vi "Application name.vi"() -> (0 "Ini file path":path, 1 "download site":string, 2 "help site":string, 3 "application name":string)   [LabVIEW 2010]
panel:
  out "Callers' Names":string[](array[string])
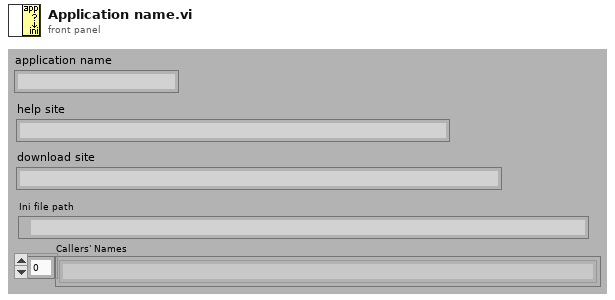
[diagram p1: front panel]
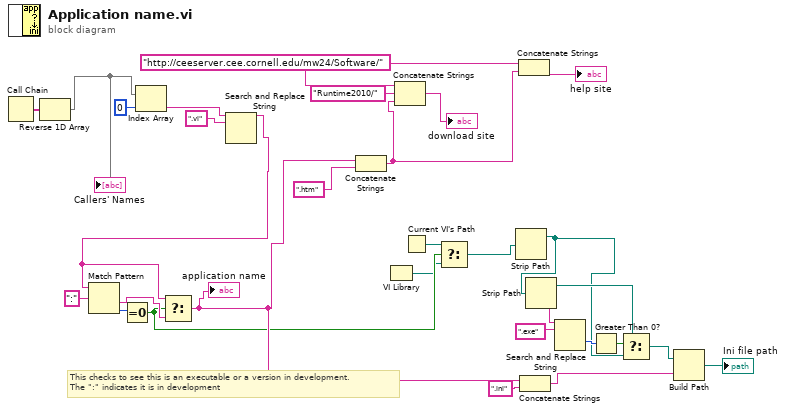
[diagram p0: block diagram]
diagram:
  w24 = "http://ceeserver.cee.cornell.edu/mw24/Software/"
  # "This checks to see this is an executable or a version in development.\nThe \":\" indicates it is in development"
  n1 = Call Chain() -> (call chain=w11:string[])
  n2 = Reverse 1D Array(array=w11) -> (reversed array=w10:string[])
  "Callers' Names" <- w10
  n3 = Index Array(array=w10, index=0) -> (element=w28:string)
  n4 = Search and Replace String(input string=w28, search string=".vi" ("replace string (\"\")")) -> (result string=w6:string)  [unwired: 6 in, 3 out]
  n5 = Match Pattern(string=w6, regular expression=":") -> (after substring=w7:string, offset past match=w8:i32)  [unwired: 1 in, 2 out]
  n6 = Equal To 0?(x=w8) -> (x = 0?=w4:bool)
  n7 = Select(t=w6, s=w4, f=w7) -> (s? t:f=w5:string)
  "application name" <- w5
  n8 = Concatenate Strings(w5, ".htm" ("replace string (\"\")")) -> (w22:string)
  n9 = VI Library() -> (path=w1:path)
  n10 = Concatenate Strings(w24, "Runtime2010/" ("string"), w22) -> (→"download site":string)
  n11 = Current VI's Path() -> (path=w3:path)
  n12 = Select(t=w3, s=w4, f=w1) -> (s? t:f=w2:path)
  n13 = Strip Path(path=w2) -> (stripped path=w16:path)  [unwired: 1 out]
  n14 = Concatenate Strings(w24, w22) -> (→"help site":string)
  n15 = Concatenate Strings(w5, ".ini") -> (w13:string)
  n16 = Strip Path(path=w16) -> (stripped path=w17:path, name=w21:string)
  n17 = Search and Replace String(input string=w21, search string=".exe") -> (offset past replacement=w19:i32)  [unwired: 6 in, 3 out]
  n18 = Greater Than 0?(x=w19) -> (x > 0?=w18:bool)
  n19 = Select(t=w17, s=w18, f=w16) -> (s? t:f=w14:path)
  n20 = Build Path(base path=w14, name or relative path=w13) -> (appended path=→"Ini file path":path)
